vi "IV_curve.vi"() -> ()   [LabVIEW 2015]
panel:
  in  "Vmin":dbl
  in  "MaxV":dbl
  in  "Gain":dbl
  in  "V to V":dbl
  out "XY Graph":T1(graph)
  out "V array out (pA)":dbl[](array[numeric])
  out "I array out (pA)":dbl[](array[numeric])
  out "Best Linear Fit":dbl[](array[numeric])
  in  "dV":dbl
  in  "Stop":bool
  in  "Dwell Time (ms)":u32
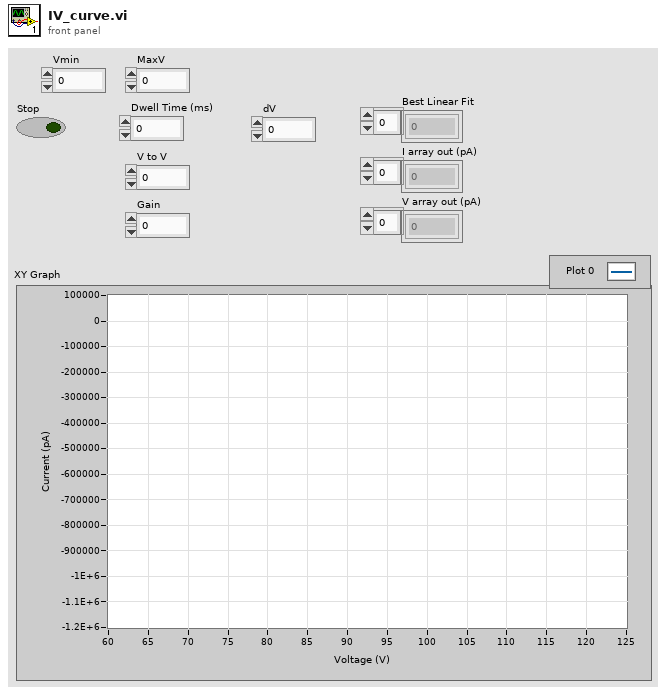
[diagram p1: front panel]
types:
  T1 = cluster{"V array out (V)":dbl[], "Best Linear Fit":dbl[]}[]
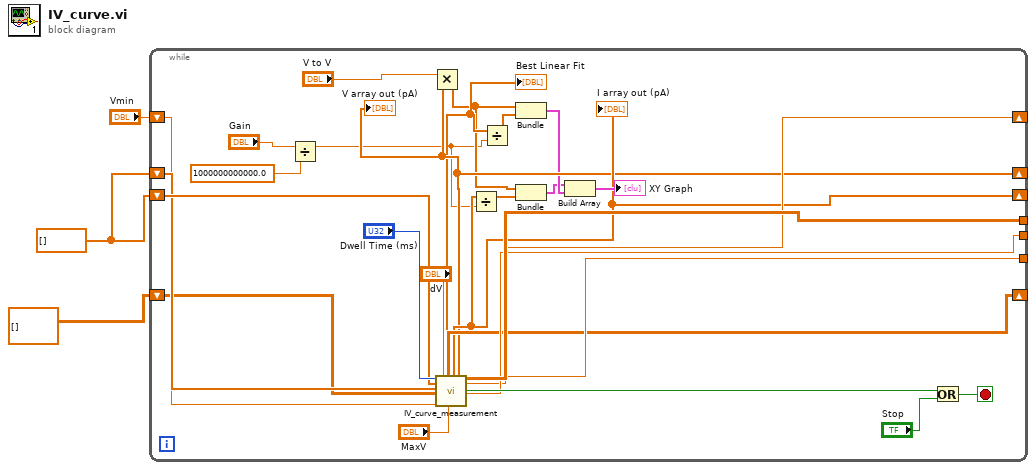
[diagram p0: block diagram]
diagram:
  w2 = dbl[] [] ("V array in (V)")
  n1 = while {
    tunnel: [w27] -> _
    tunnel: [w26] -> _
    tunnel: [w25] -> _
    shift-right: [w16] -> _
    shift-left: w2 -> [w23]
    shift-right: [w15] -> _
    shift-left: w2 -> [w22]
    shift-right: [w21] -> _
    shift-left: dbl[][] [] ("Collected array in") -> [w20]
    shift-right: [w18] -> _
    shift-left: "Vmin" -> [w17]
    stop <- w30 stop-if-true
    n2 = Divide(x="Gain", y=1000000000000.0) -> (x/y=w6:dbl)
    n3 = call "IV_curve_measurement.vi"("Dwell Time (ms)"="Dwell Time (ms)", "V array in (V)"=w23, "I array in (A)"=w22, "Collected array in"=w20, "Set V"=w17, "dV"="dV", "MaxV"="MaxV") -> ("Best Linear Fit"=w12:dbl[], "appended array"=w21:dbl[][], "I array out (pA)"=w16:dbl[], "Boolean"=w29:bool, "V array out (V)"=w15:dbl[], "intercept 2"=w25:dbl, "Collected array out"=w27:dbl[][], "Vout"=w18:dbl, "slope 2"=w26:dbl)  [unwired: 4 in]
    "Best Linear Fit" <- w12
    "I array out (pA)" <- w16
    "V array out (pA)" <- w15
    n4 = Multiply(x="V to V", y=w15) -> (x*y=w9:dbl[])
    n5 = Divide(x=w16, y=w6) -> (x/y=w13:dbl[])
    n6 = Divide(x=w12, y=w6) -> (x/y=w10:dbl[])
    n7 = Bundle(w9, w10) -> (w8:cluster{dbl[], dbl[]})  [unwired: 1 in]
    n8 = Bundle(w9, w13) -> (w7:cluster{dbl[], dbl[]})  [unwired: 1 in]
    n9 = Build Array(w7, w8) -> (→"XY Graph":cluster{dbl[], dbl[]}[])
    n10 = Or(x=w29, y="Stop") -> (x .or. y?=w30:bool)
  }
